vi "Test Ramp Field X.vi"(8 "error in (no error)":errorcluster, 9 "Target Field Rate (T/min)":dbl=0.05 format="%#_13g", 10 "Target Field (T)":dbl=0.05 format="%#_13g", 11 "Instrument.OxfordVRM in":refnum<class "Instrument.OxfordVRM.lvclass">) -> (0 "error out":errorcluster, 3 "Instrument.OxfordVRM out":refnum<class "Instrument.OxfordVRM.lvclass">)   [LabVIEW 2016, in "Instrument.OxfordVRM.lvclass"]
uses:
  Instrument.OxfordVRM.lvclass
  <vilib>/addons/_JKI Toolkits/Caraya/classes/Assert/Assert Not Error.vi
  <vilib>/addons/_JKI Toolkits/Caraya/classes/Assert/Assert Equal Value and Type_Variant.vi
  <vilib>/addons/_JKI Toolkits/Caraya/classes/Test/Test.lvclass
  <vilib>/addons/_JKI Toolkits/Caraya/classes/Assert/Assert.lvclass
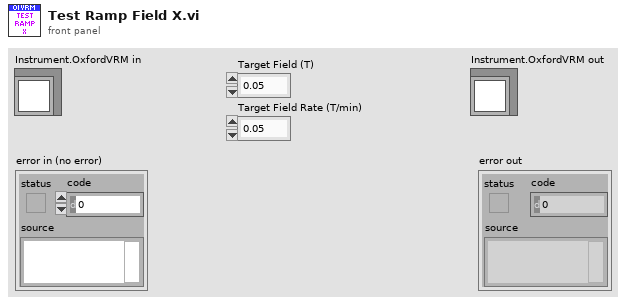
[diagram p1: front panel]
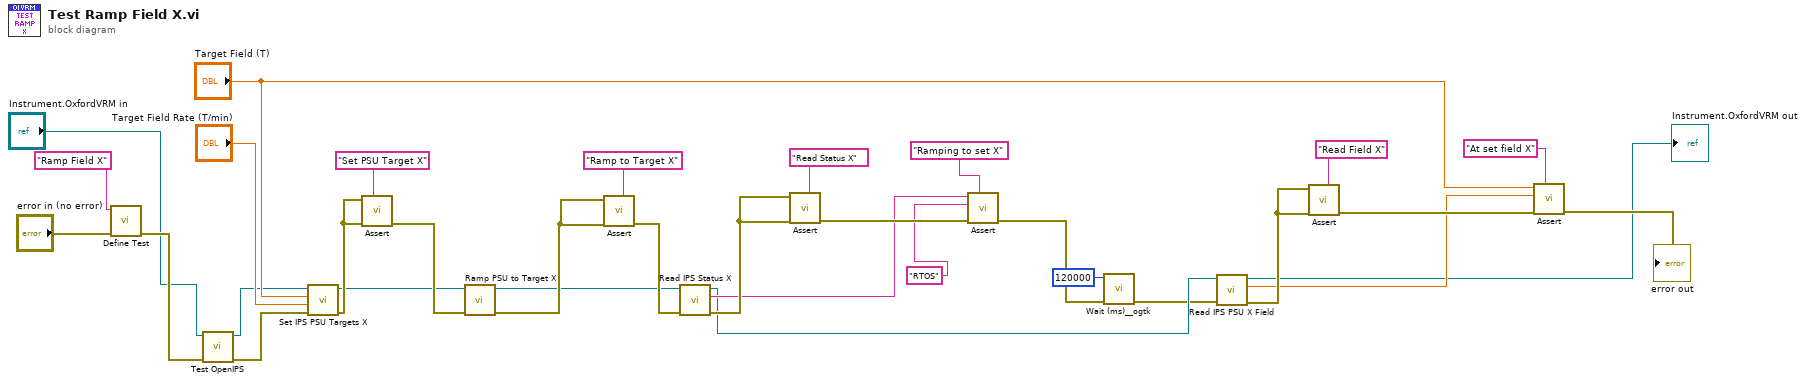
[diagram p0: block diagram]
diagram:
  n1 = call <vilib>:"Define Test.vi"("error in (no error)"="error in (no error)", "Label (VI Title)"="Ramp Field X") -> ("error out"=w4:errorcluster)  [unwired: 9 in]
  n2 = call "Test OpenIPS.vi"("error in (no error)"=w4, "Instrument.OxfordVRM in"="Instrument.OxfordVRM in") -> ("error out"=w1:errorcluster, "Instrument.OxfordVRM out"=w2:refnum<class "Instrument.OxfordVRM.lvclass">)  [unwired: 8 in]
  n3 = call "Set IPS PSU Targets X.vi"("error in (no error)"=w1, "Target Field Rate (T/min)"="Target Field Rate (T/min)", "Target Field (T)"="Target Field (T)", "Instrument.OxfordVRM in"=w2) -> ("error out"=w32:errorcluster, "Instrument.OxfordVRM out"=w21:refnum<class "Instrument.OxfordVRM.lvclass">)  [unwired: 5 in, 1 out]
  n4 = call-poly <vilib>:"Assert.vi"("Label"="Set PSU Target X", "error in (no error)"=w32, "Not Error?"=w32) -> ("error out"=w23:errorcluster)  [unwired: 8 in]
  n5 = call "Ramp PSU to Target X.vi"("error in (no error)"=w23, "Instrument.OxfordVRM in"=w21) -> ("error out"=w22:errorcluster, "Instrument.OxfordVRM out"=w19:refnum<class "Instrument.OxfordVRM.lvclass">)  [unwired: 8 in]
  n6 = call-poly <vilib>:"Assert.vi"("Label"="Ramp to Target X", "error in (no error)"=w22, "Not Error?"=w22) -> ("error out"=w20:errorcluster)  [unwired: 8 in]
  n7 = call "Read IPS Status X.vi"("error in (no error)"=w20, "Instrument.OxfordVRM in"=w19) -> ("error out"=w17:errorcluster, "Status"=w15:string, "Instrument.OxfordVRM out"=w11:refnum<class "Instrument.OxfordVRM.lvclass">)  [unwired: 7 in]
  n8 = call-poly <vilib>:"Assert.vi"("Label"="Read Status X", "error in (no error)"=w17, "Not Error?"=w17) -> ("error out"=w16:errorcluster)  [unwired: 8 in]
  n9 = call-poly <vilib>:"Assert.vi"("Label"="Ramping to set X", "error in (no error)"=w16, "Y"="RTOS", "X"=w15) -> ("error out"=w13:errorcluster)  [unwired: 7 in]
  n10 = call <userlib>:"Wait (ms)__ogtk.vi"("error in (no error)"=w13, "milliseconds to wait"=u32 120000) -> ("error out"=w10:errorcluster)  [unwired: 8 in, 1 out]
  n11 = call "Read IPS PSU X Field.vi"("error in (no error)"=w10, "Instrument.OxfordVRM in"=w11) -> ("error out"=w8:errorcluster, "Power Supply Field (T)"=w6:dbl, "Instrument.OxfordVRM out"=→"Instrument.OxfordVRM out":refnum<class "Instrument.OxfordVRM.lvclass">)  [unwired: 7 in]
  n12 = call-poly <vilib>:"Assert.vi"("Label"="Read Field X", "error in (no error)"=w8, "Not Error?"=w8) -> ("error out"=w7:errorcluster)  [unwired: 8 in]
  n13 = call-poly <vilib>:"Assert.vi"("Label"="At set field X", "error in (no error)"=w7, "Y"=w6, "X"="Target Field (T)") -> ("error out"=→"error out":errorcluster)  [unwired: 7 in]
